vi "Get_SpinProgram.vi"(8 "error in (no error)":errorcluster, 11 "SpinCoater in":refnum<class "SpinCoater.lvclass">) -> (0 "error out":errorcluster, 1 "Spin Time (s)":dbl, 2 "Spin Program":dbl[][](array[numeric]), 3 "SpinCoater out":refnum<class "SpinCoater.lvclass">)   [LabVIEW 2020, in "SpinCoater.lvclass"]
uses:
  <instrlib>/Classes/SpinCoater/SpinCoater.lvclass
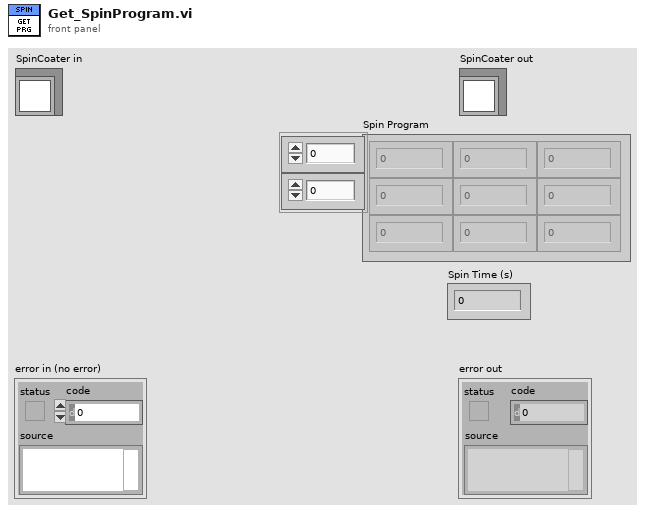
[diagram p1: front panel]
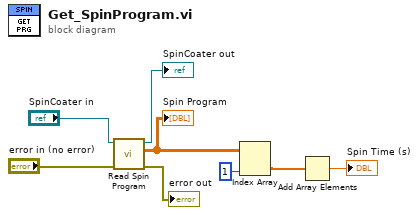
[diagram p0: block diagram]
diagram:
  n1 = call-dynamic "Read Spin Program.vi"("error in (no error)"="error in (no error)", "SpinCoater in"="SpinCoater in") -> ("error out"=→"error out":errorcluster, "Spin Program"=w3:dbl[][], "SpinCoater out"=→"SpinCoater out":refnum<class "SpinCoater.lvclass">)  [unwired: 7 in]
  "Spin Program" <- w3
  n2 = Index Array(array=w3, index (col)=1 ("index")) -> (element=w1:dbl[])  [unwired: 1 in]
  n3 = Add Array Elements(numeric array=w1) -> (sum=→"Spin Time (s)":dbl)
